vi "AlliGator Phasor Ratio Reference String.vi"(8 "error in (no error)":errorcluster, 11 "Reference #":i32) -> (0 "Error Out":errorcluster, 3 "Message":string)   [LabVIEW 2021, in "AlliGator Phasor Ratio.lvlib"]
doc: "Builds phasor reference output string."
uses:
  AlliGator Phasor Ratio.lvlib
  Phasor/Phasor.lvlib
panel:
  # "see the AlliGator License on the block diagram (Ctrl+E or Window:Show Block Diagram)"
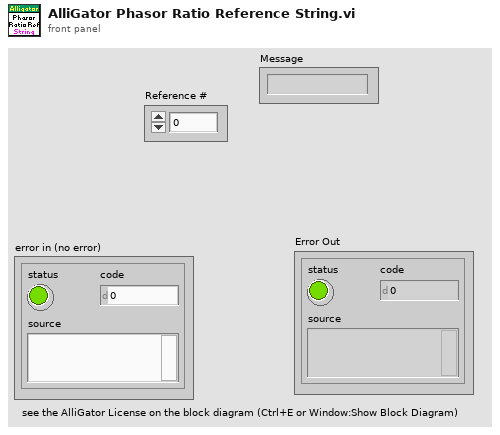
[diagram p1: front panel]
types:
  T1 = typedef "Phasor.lvlib/Phasor (g, s).ctl" = cluster{"g":dbl, "s":dbl}
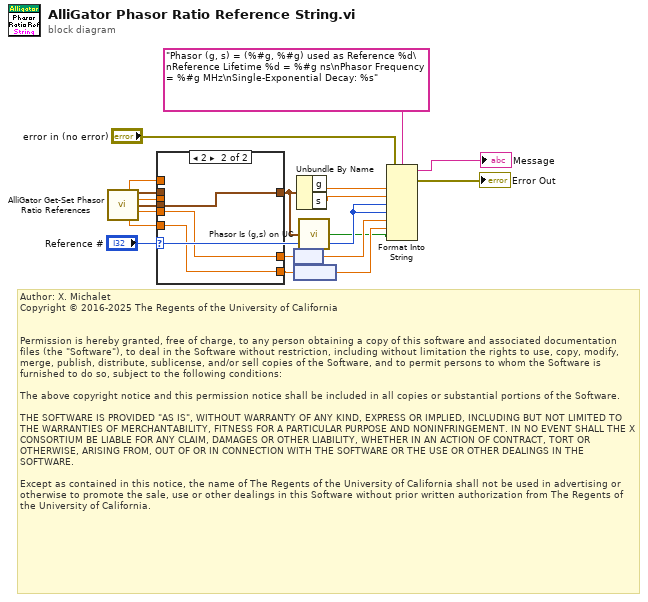
[diagram p0: block diagram]
diagram:
  # "Author: X. Michalet\nCopyright © 2016-2025 The Regents of the University of California\n \n\nPermission is hereby granted, free of charge, to any person obtaining a copy of this software and associated documentation files (the \"Software\"), to deal in the Software without restriction, including without limitation the rights to use, copy, modify, merge, publish, distribute, sublicense, and/or sell copies of the Software, and to permit persons to whom the Software is furnished to do so, subject to the following conditions:\n\nThe above copyright notice and this permission notice shall be included in all copies or substantial portions of the Software.\n\nTHE SOFTWARE IS PROVIDED \"AS IS\", WITHOUT WARRANTY OF ANY KIND, EXPRESS OR IMPLIED, INCLUDING BUT NOT LIMITED TO THE WARRANTIES OF MERCHANTABILITY, FITNESS FOR A PARTICULAR PURPOSE AND NONINFRINGEMENT. IN NO EVENT SHALL THE X CONSORTIUM BE LIABLE FOR ANY CLAIM, DAMAGES OR OTHER LIABILITY, WHETHER IN AN ACTION OF CONTRACT, TORT OR OTHERWISE, ARISING FROM, OUT OF OR IN CONNECTION WITH THE SOFTWARE OR THE USE OR OTHER DEALINGS IN THE SOFTWARE.\n\nExcept as contained in this notice, the name of The Regents of the University of California shall not be used in advertising or otherwise to promote the sale, use or other dealings in this Software without prior written authorization from The Regents of the University of California."
  n1 = call "AlliGator Get-Set Phasor Ratio References.vi"() -> ("Reference Frequency 1"=w5:dbl[unit], "Reference Phasor 1"=w13:T1, "Reference Lifetime 1"=w11:dbl[unit], "Reference Phasor 2"=w10:T1, "Reference Lifetime 2"=w9:dbl[unit], "Reference Frequency 2"=w6:dbl[unit])  [unwired: 8 in, 2 out]
  n2 = case shown="2" "Reference #" {
    tunnel: w13 -> [w22 _]
    tunnel: [w22 w23] -> w2
    tunnel: [w21 w25] -> w12
    tunnel: w11 -> [w21 _]
    tunnel: w10 -> [_ w23]
    tunnel: w9 -> [_ w25]
    tunnel: w6 -> [_ w24]
    tunnel: w5 -> [w20 _]
    tunnel: [w20 w24] -> w4
    frame 1, Default {
    }
    frame 2 {
    }
  }
  n3 = node(w12) -> (w15:dbl)
  n4 = node(w4) -> (w3:dbl)
  n5 = Unbundle By Name(w2) -> ("g"=w8:dbl, "s"=w7:dbl)
  n6 = call "Phasor Is (g,s) on UC.vi"("Phasor (g, s)"=w2) -> ("Is on UC?"=w1:bool)  [unwired: 8 in]
  n7 = Format Into String(format string="Phasor (g, s) = (%#g, %#g) used as Reference %d\nReference Lifetime %d = %#g ns\nPhasor Frequency = %#g MHz\nSingle-Exponential Decay: %s", error in="error in (no error)", w8, w7, "Reference #", "Reference #", w15, w3, w1) -> (resulting string=→"Message":string, error out=→"Error Out":errorcluster)  [unwired: 1 in]
